vi "Test1.vi"() -> ()   [LabVIEW 2017]
uses:
  <vilib>/addons/InsightCM/Devices/Shared/Common/TrendAlarm/controls/TransitionCache.ctl
  <vilib>/addons/InsightCM/MessageBus/Base/controls/TrendAlarmTransition.ctl
  <vilib>/addons/InsightCM/MessageBus/Base/controls/KeyValuePair.ctl
  <vilib>/addons/InsightCM/MessageBus/Base/controls/TrendAlarmRule.ctl
  <vilib>/addons/InsightCM/MessageBus/Base/controls/TrendAlarmLevel.ctl
  <vilib>/addons/InsightCM/MessageBus/Base/controls/AlarmAction.ctl
  <vilib>/addons/InsightCM/Devices/Shared/Common/TrendAlarm/TrendAlarm.lvlib
panel:
  out "Numeric":i32
  out "indexs":i32[](array[numeric])
  out "Array":i32[](array[numeric])
  out "cache":T1
  out "array":dbl[](array[numeric])
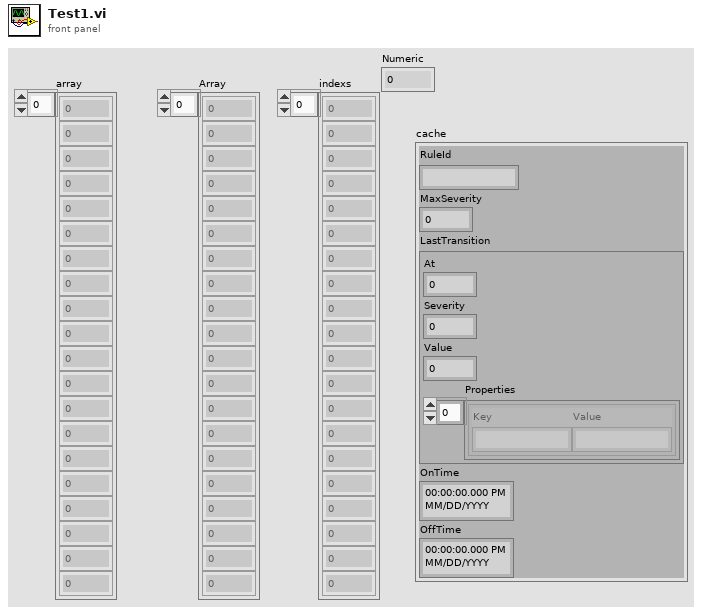
[diagram p1: front panel]
types:
  T1 = typedef "TrendAlarm.lvlib/TransitionCache.ctl" = cluster{"RuleId":string, "MaxSeverity":i32, "LastTransition":T2, "OnTime":timestamp, "OffTime":timestamp}
  T2 = typedef "TrendAlarmTransition.ctl" = cluster{"At":i64, "Severity":i32, "Value":dbl, "Properties":T3[]}
  T3 = typedef "KeyValuePair.ctl" = cluster{"Key":string, "Value":string}
  T4 = typedef "TrendAlarmRule.ctl" = cluster{"Id":string, "AssetNodeId":string, "TrendId":string, "Disabled":bool, "OperatingState":string, "Operator":string, "Hysteresis":dbl, "OnDelaySeconds":dbl, "OffDelaySeconds":dbl, "Levels":T5[], "Properties":T3[]}
  T5 = typedef "TrendAlarmLevel.ctl" = cluster{"Severity":i32, "CompareTo":dbl, "Actions":T6[]}
  T6 = typedef "AlarmAction.ctl" = cluster{"Type":string, "Props":T3[]}
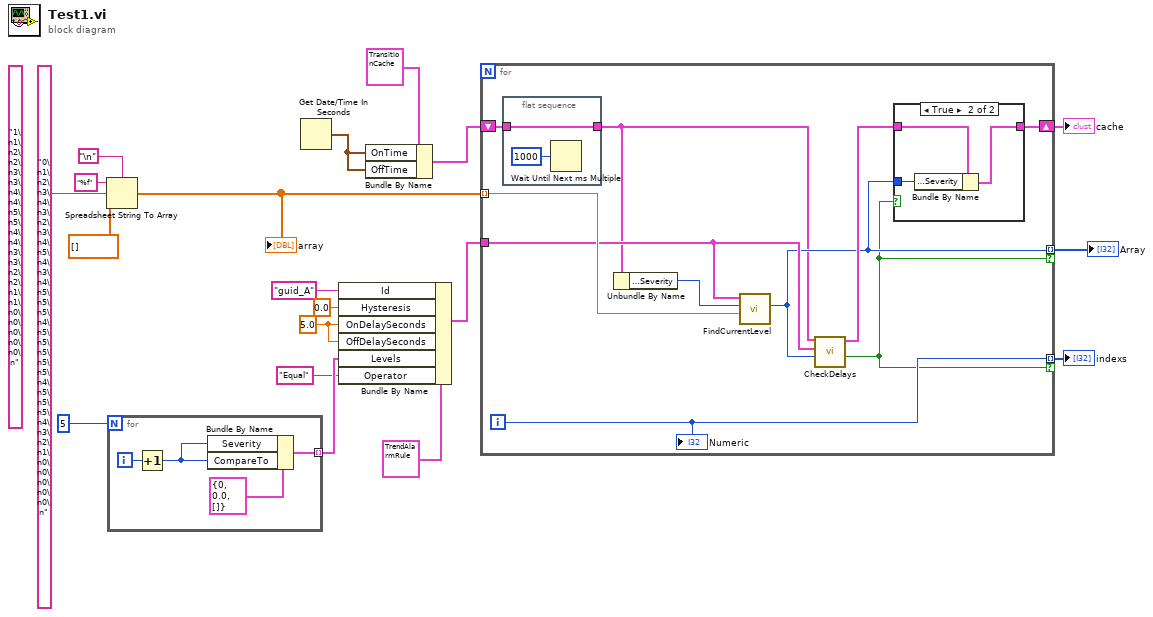
[diagram p0: block diagram]
diagram:
  (unwired) "1\n1\n2\n2\n3\n3\n4\n4\n5\n5\n4\n4\n3\n3\n2\n2\n1\n1\n0\n0\n0\n0\n0\n"
  w11 = 5.0 ("OnDelaySeconds")
  n1 = Spreadsheet String To Array(delimiter (Tab)="\n", format string="%f", spreadsheet string="0\n1\n2\n3\n4\n3\n2\n3\n4\n5\n4\n3\n4\n5\n5\n5\n4\n5\n5\n5\n5\n5\n4\n5\n5\n5\n4\n3\n2\n1\n0\n0\n0\n0\n0\n", array type (2D Dbl)=dbl[] []) -> (array=w16:dbl[])
  "array" <- w16
  n2 = for {
    N: 5 -> [_]
    tunnel: [w20] -> w9 mode=indexing
    i -> [w22]
    n3 = Increment(x=w22) -> (x+1=w21:i32)
    n4 = Bundle By Name(cluster=T5 {"Severity"=0, "CompareTo"=0.0, "Actions"=[]} ("Level"), "Severity"=w21, "CompareTo"=w21) -> (w20:T5)
  }
  n5 = Get Date/Time In Seconds() -> (seconds since 1Jan1904=w1:timestamp)
  n6 = Bundle By Name(cluster=T4 {"Id"="", "AssetNodeId"="", "TrendId"="", "Disabled"=FALSE, "OperatingState"="", "Operator"="", "Hysteresis"=0.0, "OnDelaySeconds"=0.0, "OffDelaySeconds"=0.0, "Levels"=[], "Properties"=[]} ("rule"), "Id"="guid_A", "Hysteresis"=0.0, "OnDelaySeconds"=w11, "OffDelaySeconds"=w11, "Levels"=w9, "Operator"="Equal") -> (w7:T4)
  n7 = Bundle By Name(cluster=T1 {"RuleId"="", "MaxSeverity"=0, "LastTransition"={"At"=0, "Severity"=0, "Value"=0.0, "Properties"=[]}, "OnTime"=timestamp(0 s since 1904-01-01), "OffTime"=timestamp(0 s since 1904-01-01)} ("cache in"), "OnTime"=w1, "OffTime"=w1) -> (w2:T1)
  n8 = for {
    tunnel: w16 -> [w33] mode=indexing
    shift-right: [w29] -> w8
    shift-left: w2 -> [w24]
    tunnel: w7 -> [w32]
    tunnel: [w27] -> w5 mode=indexing if=w26
    tunnel: [w31] -> w4 mode=indexing if=w26
    i -> [w31]
    n9 = flat-sequence {
      tunnel: [w34] -> w25
      tunnel: w24 -> [w34]
      frame #0 {
        n10 = Wait Until Next ms Multiple(millisecond multiple=u32 1000) -> ()  [unwired: 1 out]
      }
    }
    n11 = Unbundle By Name(w25) -> ("LastTransition.Severity"=w28:i32)
    n12 = call <vilib>:"FindCurrentLevel.vi"("value"=w33, "latched severity"=w28, "rule"=w32) -> ("severity out"=w27:i32)  [unwired: 8 in]
    n13 = call <vilib>:"CheckDelays.vi"("current level"=w27, "rule"=w32, "cache in"=w25) -> ("update"=w26:bool, "cache out"=w30:T1)  [unwired: 7 in]
    n14 = case shown="True" w26 {
      tunnel: w30 -> [w36 w39]
      tunnel: [w36 w38] -> w29
      tunnel: w27 -> [_ w37]
      frame False {
      }
      frame True {
        n15 = Bundle By Name(cluster=w39, "LastTransition.Severity"=w37) -> (w38:T1)
      }
    }
    "Numeric" <- w31
  }
  "cache" <- w8
  "Array" <- w5
  "indexs" <- w4
